vi "CPT-Compute PTC.vi"(0 "Mag":dbl[][](array[numeric]), 5 "Phase":dbl[][](array[numeric]), 7 "df (Hz)":dbl, 9 "Cal mic index":i32, 11 "error in (no error)":errorcluster, 12 "Cal Mic Sensitivity \n(dB V/SPL)":dbl=-151.3710301348461 format="%.2f", 13 "Cal Mic Gain (dB)":dbl=20.0, 14 "Probe Mic Gain (dB)":dbl=20.0) -> (4 "PTC Mag":dbl[](array[numeric]), 6 "PTC Phase":dbl[](array[numeric]), 8 "Frequency":dbl[](array[numeric]), 15 "error out":errorcluster)   [LabVIEW 2020]
uses:
  epl-vi-lib/Utility VIs/Math VIs/LinSpace (x0-dx-npts).vi
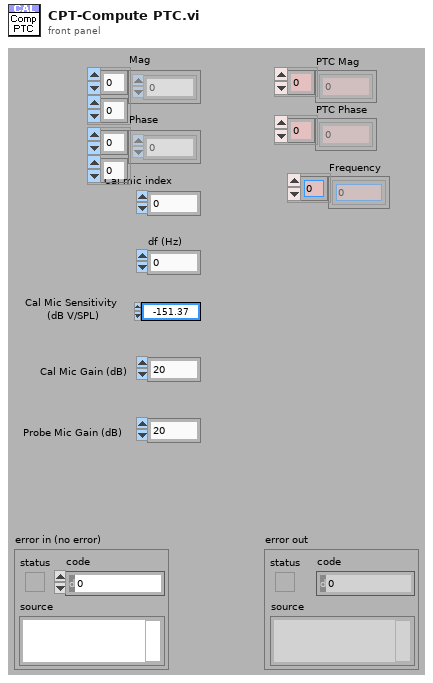
[diagram p1: front panel]
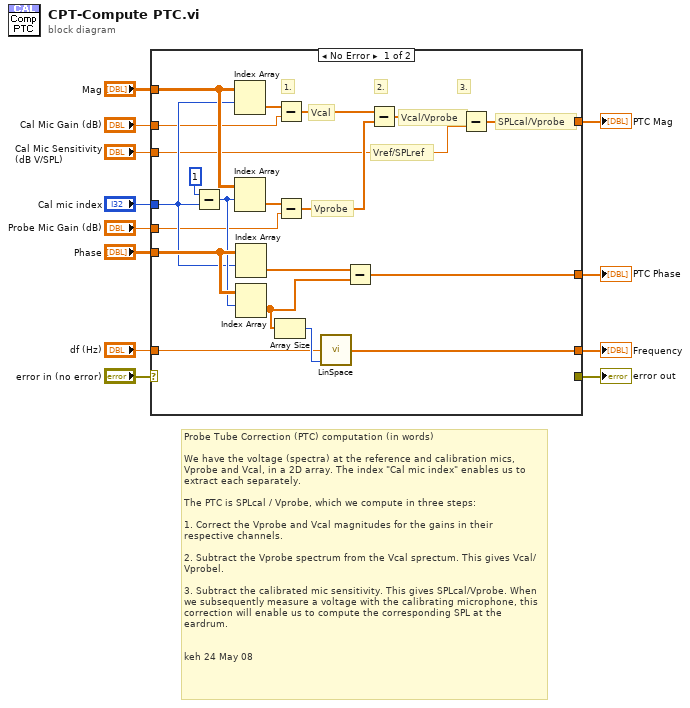
[diagram p0: block diagram]
diagram:
  # "Probe Tube Correction (PTC) computation (in words)\n\nWe have the voltage (spectra) at the reference and calibration mics, Vprobe and Vcal, in a 2D array. The index \"Cal mic index\" enables us to extract each separately. \n\nThe PTC is SPLcal / Vprobe, which we compute in three steps:\n\n1. Correct the Vprobe and Vcal magnitudes for the gains in their respective channels.\n\n2. Subtract the Vprobe spectrum from the Vcal sprectum. This gives Vcal/Vprobel.\n\n3. Subtract the calibrated mic sensitivity. This gives SPLcal/Vprobe. When we subsequently measure a voltage with the calibrating microphone, this correction will enable us to compute the corresponding SPL at the eardrum.\n\n\nkeh 24 May 08"
  n1 = case shown="No Error" "error in (no error)" {
    selector: "error in (no error)" -> [_ w33]
    tunnel: "Mag" -> [w31 _]
    tunnel: "Phase" -> [w30 _]
    tunnel: [w13 _] -> w10
    tunnel: [w27 _] -> w9
    tunnel: [w25 _] -> w8
    tunnel: "df (Hz)" -> [w24 _]
    tunnel: [_ w33] -> w5
    tunnel: "Cal mic index" -> [w22 _]
    tunnel: "Cal Mic Gain (dB)" -> [w19 _]
    tunnel: "Probe Mic Gain (dB)" -> [w17 _]
    tunnel: "Cal Mic Sensitivity \n(dB V/SPL)" -> [w14 _]
    frame No Error {
      # "Vref/SPLref"
      # "SPLcal/Vprobe"
      # "Vcal/Vprobe"
      # "Vprobe"
      # "Vcal"
      # "3."
      # "2."
      # "1."
      n2 = Subtract(x=1, y=w22) -> (x-y=w29:i32)
      n3 = Index Array(array=w31, index (row)=w22) -> (element=w20:dbl[])  [unwired: 1 in]
      n4 = Index Array(array=w31, index (row)=w29) -> (element=w18:dbl[])  [unwired: 1 in]
      n5 = Index Array(array=w30, index (row)=w22) -> (element=w28:dbl[])  [unwired: 1 in]
      n6 = Index Array(array=w30, index (row)=w29) -> (element=w23:dbl[])  [unwired: 1 in]
      n7 = Array Size(array=w23) -> (size(s)=w26:i32)
      n8 = Subtract(x=w20, y=w19) -> (x-y=w21:dbl[])
      n9 = Subtract(x=w18, y=w17) -> (x-y=w16:dbl[])
      n10 = call-poly "LinSpace.vi"("npts"=w26, "dx"=w24) -> ("Array"=w25:dbl[])  [unwired: 2 in, 1 out]
      n11 = Subtract(x=w28, y=w23) -> (x-y=w27:dbl[])
      n12 = Subtract(x=w21, y=w16) -> (x-y=w15:dbl[])
      n13 = Subtract(x=w15, y=w14) -> (x-y=w13:dbl[])
    }
    frame Error {
    }
  }
  "PTC Mag" <- w10
  "PTC Phase" <- w9
  "Frequency" <- w8
  "error out" <- w5
